vi "Open Hardware.vi"(8 "error in (no error)":errorcluster, 11 "Instrument.Template in":refnum<class "Instrument.Element2.lvclass">) -> (0 "error out":errorcluster, 3 "Instrument.Template out":refnum<class "Instrument.Element2.lvclass">)   [LabVIEW 2019, in "Instrument.Element2.lvclass"]
uses:
  Instrument.Element2.lvclass
  <vilib>/Instr/_visa.llb/VISA Configure Serial Port (Instr).vi
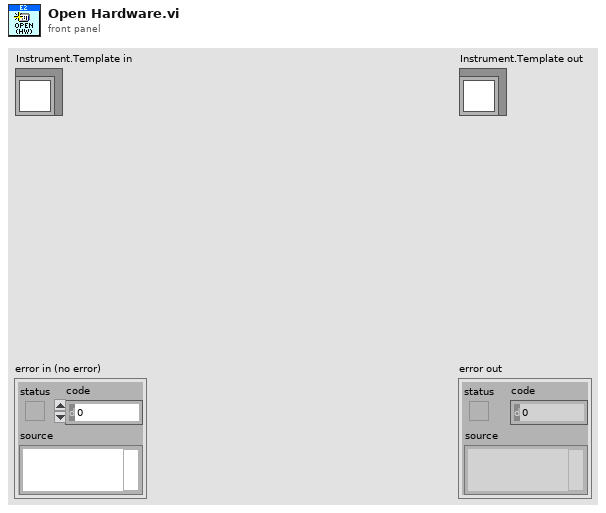
[diagram p1: front panel]
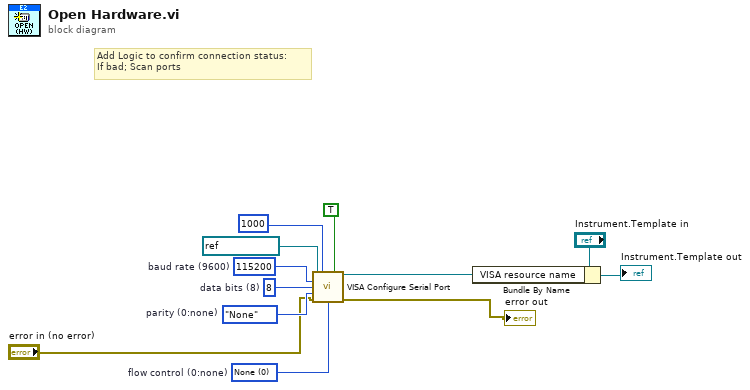
[diagram p0: block diagram]
diagram:
  w5 = u16 0 items=["None", "XON/XOFF", "RTS/CTS", "XON/XOFF & RTS/CTS", "DTR/DSR", "XON/XOFF & DTR/DSR"]  # flow control (0:none)
  w6 = u16 8  # data bits (8)
  w7 = u32 115200  # baud rate (9600)
  w8 = enum16{"None", "Odd", "Even", "Mark", "Space"}."None"  # parity (0:none)
  # "Add Logic to confirm connection status:\nIf bad; Scan ports"
  n1 = call-poly "VISA Configure Serial Port"("VISA resource name"=refnum<visa-resource-name> "Element2" ("Resource Name"), "timeout (10sec)"=u32 1000, "Enable Termination\nChar (T)"=TRUE ("Enable Termination\nChar (T)"), "baud rate (9600)"=w7, "data bits (8)"=w6, "parity (0:none)"=w8, "error in (no error)"="error in (no error)", "flow control (0:none)"=w5) -> ("VISA resource name out"=w3:refnum<visa-resource-name>, "error out"=→"error out":errorcluster)  [unwired: 6 out]
  n2 = Bundle By Name(cluster="Instrument.Template in", "VISA resource name"=w3) -> (→"Instrument.Template out":refnum<class "Instrument.Element2.lvclass">)
